vi "FC_Test_Get_Team_Attribute.vi"() -> ()   [LabVIEW 2014]
uses:
  FC_Target.ctl
  FC_FIRST Client.lvlib
panel:
  out "Team Data Cluster":T1
  in  "Team # (Ex: 1)":string="1"
  # "This VI demonstrates getting the attributes of a team"
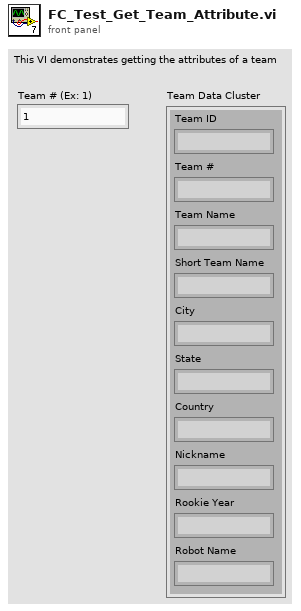
[diagram p1: front panel]
types:
  T1 = cluster{"Team ID":string, "Team #":string, "Team Name":string, "Short Team Name":string, "City":string, "State":string, "Country":string, "Nickname":string, "Rookie Year":string, "Robot Name":string}
  T2 = typedef "FC_FIRST Client.lvlib/FC_Target.ctl" = enum16{"Teams", "Competitions"}
  T3 = typedef "FC_FIRST Client.lvlib/FC_Team Attributes.ctl" = cluster{"Team ID":string, "Team #":string, "Team Name":string, "Short Team Name":string, "City":string, "State":string, "Country":string, "Nickname":string, "Rookie Year":string, "Robot Name":string}
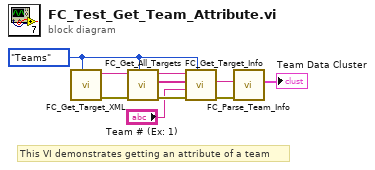
[diagram p0: block diagram]
diagram:
  w6 = FC_Target."Teams" ("Enum")
  # "This VI demonstrates getting an attribute of a team"
  n1 = call "FC_Get_Target_XML.vi"("Target"=w6) -> ("error out"=w7:errorcluster, "All Teams XML"=w10:string)  [unwired: 9 in]
  n2 = call "FC_Get_All_Targets.vi"("Target"=w6, "Error In"=w7, "Target XML"=w10) -> ("error out"=w8:errorcluster, "Array of Targets"=w5:string[], "Copy of Target XML"=w9:string)  [unwired: 6 in]
  n3 = call "FC_Get_Target_Info.vi"("Target"=w6, "Error In"=w8, "Desired Target"="Team # (Ex: 1)", "Array of Targets"=w5, "Target XML"=w9) -> ("error out"=w2:errorcluster, "Target Info"=w3:string)  [unwired: 5 in]
  n4 = call "FC_Parse_Team_Info.vi"("Error In"=w2, "All Team Data"=w3) -> ("Team Data Cluster"=→"Team Data Cluster":T3)  [unwired: 8 in, 1 out]
